vi "Read Position Left.vi"(8 "error in (no error)":errorcluster, 11 "GObject.lvclass in":refnum<class "GObject.lvclass">) -> (0 "error out":errorcluster, 2 "Left":i32, 3 "GObject.lvclass out":refnum<class "GObject.lvclass">)   [LabVIEW 2015, in "GObject.lvclass"]
uses:
  GObject.lvclass
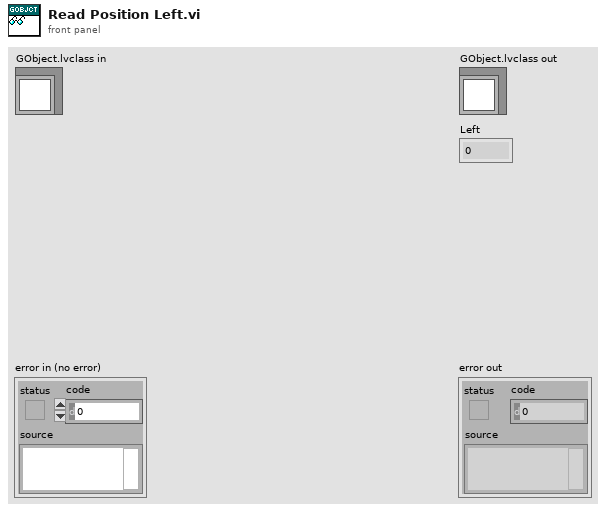
[diagram p1: front panel]
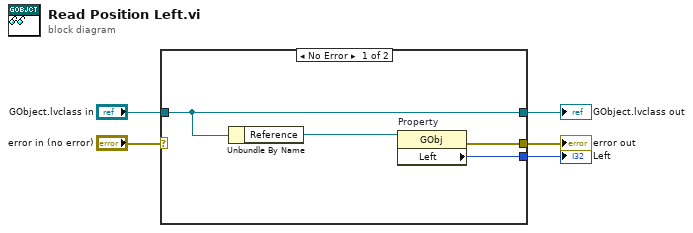
[diagram p0: block diagram]
diagram:
  n1 = case shown="No Error" "error in (no error)" {
    selector: "error in (no error)" -> [_ w11]
    tunnel: [w8 w11] -> w4
    tunnel: [w7 w10] -> w2
    tunnel: "GObject.lvclass in" -> [w7 w10]
    tunnel: [w9 _] -> w1
    frame No Error {
      n2 = Unbundle By Name(w7) -> ("Reference"=w6:refnum<vi>)
      n3 = property on="Property" class="GObj"(reference=w6) -> (error out=w8:errorcluster, "Left"=w9:i32)  [unwired: 1 in, 1 out]
    }
    frame Error {
    }
  }
  "error out" <- w4
  "GObject.lvclass out" <- w2
  "Left" <- w1
